vi "Setup FPGA - 9025.vi"(2 "Error In":errorcluster) -> (0 "Error Out":errorcluster, 1 "FPGA VI Reference Out":refnum<k20>)   [LabVIEW 2017]
uses:
  <vilib>/FPGAPlugInAG/cRIO-9114/niLvFpga_Open_cRIO-9114.vi
  <vilib>/rvi/interface/common/dynamic/niFpgaDynamicAddResources.vi
  <vilib>/FPGAPlugInAG/Dynamic/niLvFpga_Run_Dynamic.vi
  <vilib>/Utility/error.llb/Error Cluster From Error Code.vi
  <vilib>/rvi/errors/niLvFpgaAdjustHostInterfaceError.vi
  <vilib>/rvi/interface/nirviOpenFPGA/nirviOpenFPGA.xnode
  FPGA Bitfiles/Project_FPGATarget_FPGAMain_G8lxl2g5ckA.lvbitx
  FPGA Main - 9025.vi
  <vilib>/rvi/interface/nirviMethod/nirviMethod.xnode
  <vilib>/rvi/interface/nirviReadWriteControl/nirviReadWriteControl.xnode
  NiFpgaLv.dll
  <vilib>/rvi/interface/Simulation/niFpgaSimulationCallBeginRW.vi
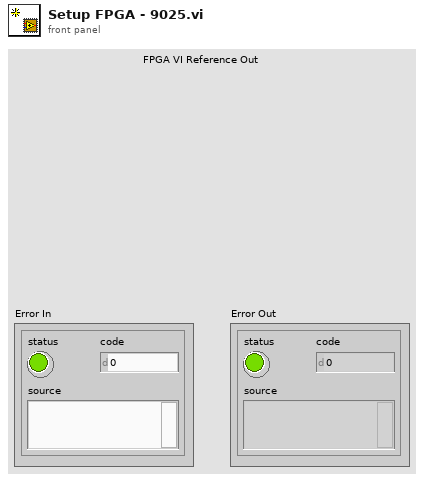
[diagram p1: front panel]
types:
  T1 = cluster{"TC Low Speed Logging":u32, "TC  High Speed Logging":u32, "PS Low Speed Logging":u32, "PS  High Speed Logging":u32, "LC Low Speed Logging":u32, "LC  High Speed Logging":u32}
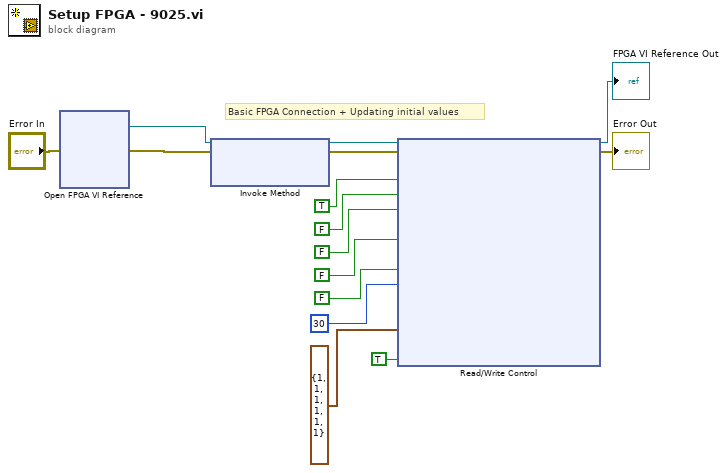
[diagram p0: block diagram]
diagram:
  # "Basic FPGA Connection + Updating initial values"
  n1 = xnode "Open FPGA VI Reference"("error in"="Error In") -> ("FPGA VI Reference Out"=w5:refnum<k20>, "error out"=w4:errorcluster)  [unwired: 1 in]
  n2 = xnode "Invoke Method"("FPGA VI Reference In"=w5, "error in"=w4) -> ("FPGA VI Reference Out"=w14:refnum<k20>, "error out"=w13:errorcluster)  [unwired: 1 in]
  n3 = xnode "Read/Write Control"("FPGA VI Reference In"=w14, "error in"=w13, "Manual Mode"=TRUE, "Start Automated Sequence"=FALSE, "Emergency Shutdown"=FALSE, "High Speed?"=FALSE, "Logging?"=FALSE, "Poll Rate"=u32 30, "Logging Settings"=T1 {"TC Low Speed Logging"=1, "TC  High Speed Logging"=1, "PS Low Speed Logging"=1, "PS  High Speed Logging"=1, "LC Low Speed Logging"=1, "LC  High Speed Logging"=1}, "Emergency Normally Open/Closed"=TRUE) -> ("FPGA VI Reference Out"=→"FPGA VI Reference Out":refnum<k20>, "error out"=→"Error Out":errorcluster)  [unwired: 1 in, 5 out]
